vi "Ref data LV2.vi"() -> ()   [LabVIEW 2020]
uses:
  Typedefs/Cluster data.ctl
panel:
  out "Output Refnum":refnum<user-event>
  in  "error in":errorcluster
  in  "Enum":T1(ring)
  in  "Data":T2
  out "error out":errorcluster
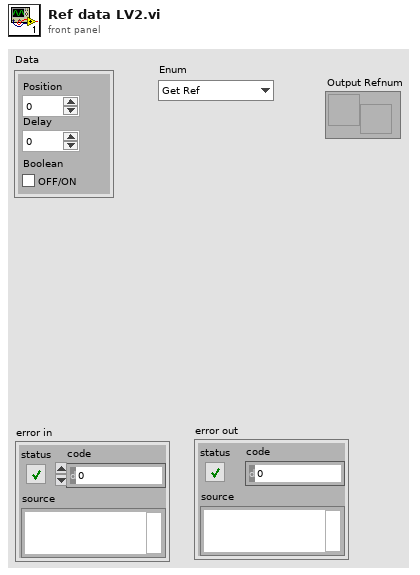
[diagram p1: front panel]
types:
  T1 = enum16{"Get Ref", "Destroy", "Create", "Generate"}
  T2 = typedef "Cluster data.ctl" = cluster{"Position":dbl, "Delay":dbl, "Boolean":bool}
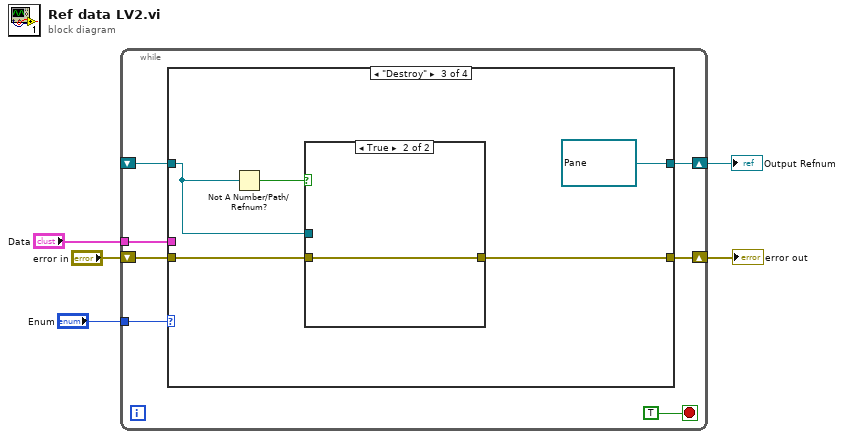
[diagram p0: block diagram]
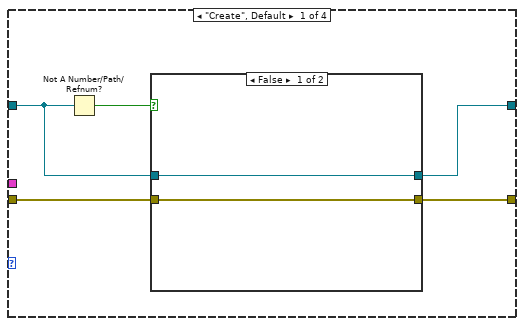
[diagram p2: hidden frame]
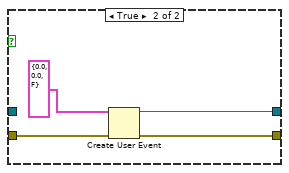
[diagram p3: hidden frame]
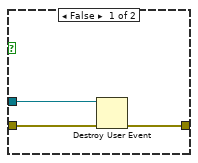
[diagram p5: hidden frame]
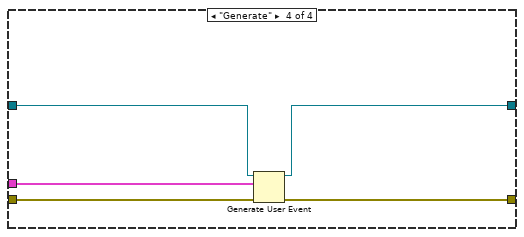
[diagram p6: hidden frame]
diagram:
  n1 = while {
    tunnel: "Enum" -> [w12]
    tunnel: "Data" -> [w11]
    shift-right: [w9] -> w2
    shift-left: "error in" -> [w10]
    shift-right: [w6] -> w1
    shift-left: _ -> [w7]
    stop <- TRUE stop-if-true
    n2 = case shown="\"Destroy\"" w12 {
      tunnel: [w17 w24 w29 w38] -> w9
      tunnel: w10 -> [w16 w24 w30 w39]
      tunnel: [w15 w25 refnum<user-event> refnum ("Data") w36] -> w6
      tunnel: w7 -> [w13 w25 w28 w35]
      tunnel: w11 -> [_ _ _ w37]
      frame "Create", Default {
        n3 = Not A Number/Path/Refnum?(number/path/refnum=w13) -> (NaN/Path/Refnum?=w14:bool)
        n4 = case shown="False" w14 {
          tunnel: [w19 w23] -> w17
          tunnel: w16 -> [w19 w22]
          tunnel: [w18 w21] -> w15
          tunnel: w13 -> [w18 _]
          frame False {
          }
          frame True {
            n5 = Create User Event(user event datatype=T2 {"Position"=0.0, "Delay"=0.0, "Boolean"=FALSE} ("Data"), error in=w22) -> (user event=w21:refnum<user-event>, error out=w23:errorcluster)
          }
        }
      }
      frame "Get Ref" {
      }
      frame "Destroy" {
        n6 = Not A Number/Path/Refnum?(number/path/refnum=w28) -> (NaN/Path/Refnum?=w27:bool)
        n7 = case shown="True" w27 {
          tunnel: w30 -> [w33 w34]
          tunnel: w28 -> [w32 _]
          tunnel: [w31 w34] -> w29
          frame False {
            n8 = Destroy User Event(user event=w32, error in=w33) -> (error out=w31:errorcluster)
          }
          frame True {
          }
        }
      }
      frame "Generate" {
        n9 = Generate User Event(user event=w35, event data cluster=w37, error in=w39) -> (user event out=w36:refnum<user-event>, error out=w38:errorcluster)  [unwired: 1 in]
      }
    }
  }
  "error out" <- w2
  "Output Refnum" <- w1
